vi "cm_Convert State For Save.vi"(2 "Container State":T1, 3 "Display State":T2={"Chan"=[], "First Drop?"=FALSE, "Notifier Name"="", "Refresh View"=FALSE, "Scale to Input Range"=FALSE, "Linear View"=FALSE, "Display"={"Current"=6618880, "Peak"=6618880}, "Property/Method"=enum."No Update", "Time Display Ref"=[]}) -> (1 "Display State To Save":variant)   [LabVIEW 2012, in "Channel Monitor.xctl"]
uses:
  Channel Monitor.xctl
  cm_Channel Monitor State.ctl
  TypeDef/cm_Property_Method.ctl
  <vilib>/_xctls/Container State.ctl
  <vilib>/_xctls/XControlSupport.lvlib
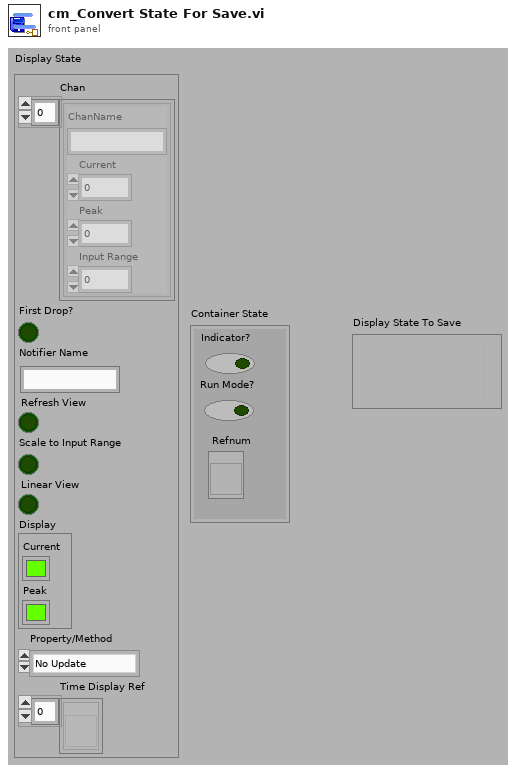
[diagram p1: front panel]
types:
  T1 = typedef "XControlSupport.lvlib/Container State.ctl" = cluster{"Indicator?":bool, "Run Mode?":bool, " Refnum":refnum<vi>}
  T2 = typedef "Channel Monitor.xctl/cm_Channel Monitor State.ctl" = cluster{"Chan":cluster{"ChanName":string, "Current":dbl, "Peak":dbl, "Input Range":dbl}[], "First Drop?":bool, "Notifier Name":string, "Refresh View":bool, "Scale to Input Range":bool, "Linear View":bool, "Display":cluster{"Current":u32, "Peak":u32}, "Property/Method":T3, "Time Display Ref":refnum<vi>[]}
  T3 = typedef "Channel Monitor.xctl/cm_Property_Method.ctl" = enum16{"No Update", "Color: Currrent", "Color: Peak", "Close Time Displays"}
  T4 = cluster{"ChanName":string, "Current":dbl, "Peak":dbl, "Input Range":dbl}[]
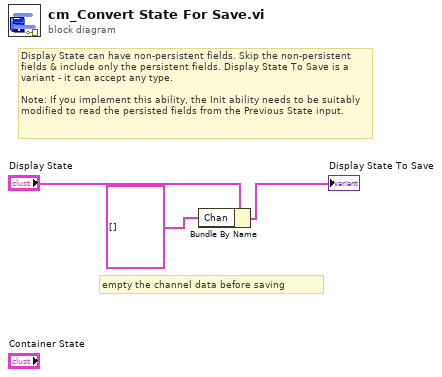
[diagram p0: block diagram]
diagram:
  # "empty the channel data before saving"
  # "Display State can have non-persistent fields. Skip the non-persistent fields & include only the persistent fields. Display State To Save is a variant - it can accept any type.\n\nNote: If you implement this ability, the Init ability needs to be suitably modified to read the persisted fields from the Previous State input."
  n1 = Bundle By Name(cluster="Display State", "Chan"=T4 []) -> (→"Display State To Save":T2)
